vi "aDeserializeMethod.vi"(0 "object in":refnum<class "JSONJKI.lvclass">, 2 "String":string, 5 "error in (no error)":errorcluster) -> (14 "object out":refnum<class "JSONJKI.lvclass">, 15 "Class":string, 16 "Method":string, 17 "Inputsstring":string, 19 "error out":errorcluster)   [LabVIEW 2018, in "JSONJKI.lvclass"]
uses:
  JSONJKI.lvclass
  <vilib>/addons/_JKI.lib/Serialization/JSON/JKI JSON Serialization.lvlib
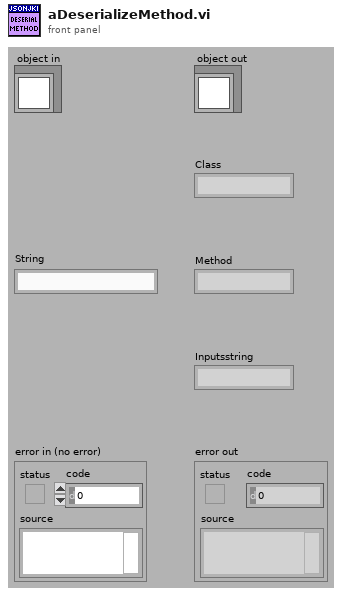
[diagram p1: front panel]
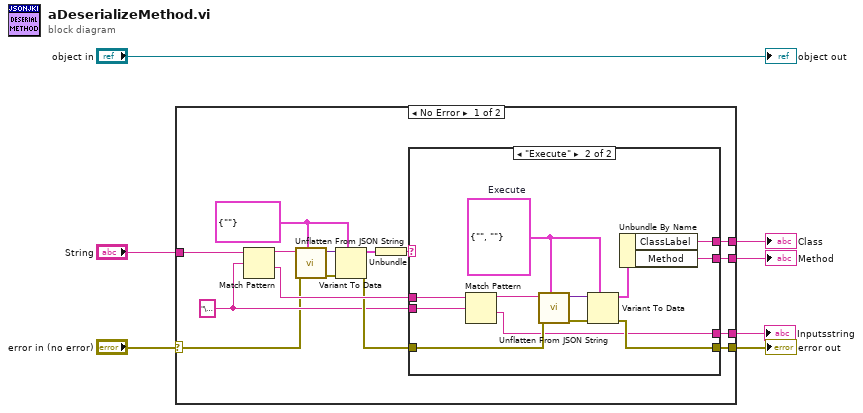
[diagram p0: block diagram]
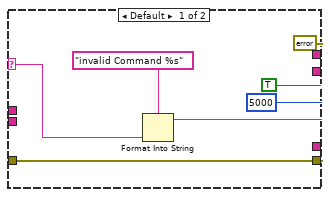
[diagram p2: hidden frame]
diagram:
  n1 = case shown="No Error" "error in (no error)" {
    selector: "error in (no error)" -> [w13 w44]
    tunnel: [w12 w44] -> w6
    tunnel: "String" -> [w14 _]
    tunnel: [w11 _] -> w2
    tunnel: [w10 _] -> w3
    tunnel: [w8 _] -> w1
    frame No Error {
      w9 = cluster{"Command":string} {"Command"=""} ("output cluster")
      w15 = "\u0017" ("Delimiter")
      n2 = Match Pattern(string=w14, regular expression=w15) -> (before substring=w19:string, after substring=w22:string)  [unwired: 1 in, 2 out]
      n3 = call <vilib>:"Unflatten From JSON String.vi"("Type and Defaults"=w9, "error in (no error)"=w13, "JSON String"=w19) -> ("error out"=w20:errorcluster, "Variant"=w21:variant)  [unwired: 7 in]
      n4 = Variant To Data(error in=w20, type=w9, Variant=w21) -> (data=w18:cluster{"Command":string}, error out=w16:errorcluster)
      n5 = Unbundle(w18) -> ("Command"=w17:string)
      n6 = case shown="\"Execute\"" w17 {
        selector: w17 -> [w27 _]
        tunnel: w22 -> [_ w39]
        tunnel: w16 -> [w30 w34]
        tunnel: w15 -> [_ w37]
        tunnel: [w31 w33] -> w12
        tunnel: [_ w36] -> w11
        tunnel: [_ w35] -> w10
        tunnel: [_ w32] -> w8
        frame Default {
          n7 = Format Into String(format string="invalid Command %s", w27) -> (resulting string=w25:string)  [unwired: 2 in, 1 out]
          n8 = Bundle By Name(cluster=errorcluster {"status"=TRUE, "code"=5000, "source"="invalid Commnad"} ("error in"), "status"=TRUE, "code"=5000, "source"=w25) -> (w26:errorcluster)
          n9 = Merge Errors(w30, w26) -> (w31:errorcluster)
        }
        frame "Execute" {
          w40 = cluster{"ClassLabel":string, "Method":string} {"ClassLabel"="", "Method"=""}  # Execute
          n10 = Match Pattern(string=w39, regular expression=w37) -> (before substring=w38:string, after substring=w32:string)  [unwired: 1 in, 2 out]
          n11 = call <vilib>:"Unflatten From JSON String.vi"("Type and Defaults"=w40, "error in (no error)"=w34, "JSON String"=w38) -> ("error out"=w43:errorcluster, "Variant"=w42:variant)  [unwired: 7 in]
          n12 = Variant To Data(error in=w43, type=w40, Variant=w42) -> (data=w41:cluster{"ClassLabel":string, "Method":string}, error out=w33:errorcluster)
          n13 = Unbundle By Name(w41) -> ("ClassLabel"=w36:string, "Method"=w35:string)
        }
      }
    }
    frame Error {
    }
  }
  "error out" <- w6
  "Class" <- w2
  "Method" <- w3
  "Inputsstring" <- w1
  "object out" <- "object in"
